vi "temperature_read.vi"(10 "T = Digital, F = Analog":bool) -> (3 "temperature array":dbl[](array[numeric]))   [LabVIEW 2021]
uses:
  <vilib>/DAQmx/read.llb/DAQmx Read (Analog 1D DBL NChan 1Samp).vi
  SmallBore_Labview/global_variables.vi
  <vilib>/DAQmx/create/channels.llb/DAQmx Create Channel (AI-Voltage-Basic).vi
  <vilib>/DAQmx/miscellaneous.llb/DAQmx Fill In Error Info.vi
panel:
  out "Thermometer 5: \nWater tank Small":dbl(slide) scale=0.0..100.0
  in  "Tab Control":enum32{"Digital", "Analog"}(tab)
  out "output array":bool[][](array[boolean])
  in  "Number of runs (>1)":i32=3
  in  "baud rate":u32=3906
  in  "No. expected bits":u16=64
  out "data":dbl[](array[numeric]) format="%0.2f"
  in  "milliseconds to wait":u32=100
  out "Thermometer 4: \nWater tank Big":dbl(slide) scale=0.0..100.0
  out "Thermometer 3: \nTx Filt Xfmer":dbl(slide) scale=0.0..100.0
  out "Thermometer 2: \nTx Filt L6":dbl(slide) scale=0.0..100.0
  out "Thermometer 1: \nTx Filt L7":dbl(slide) scale=0.0..100.0
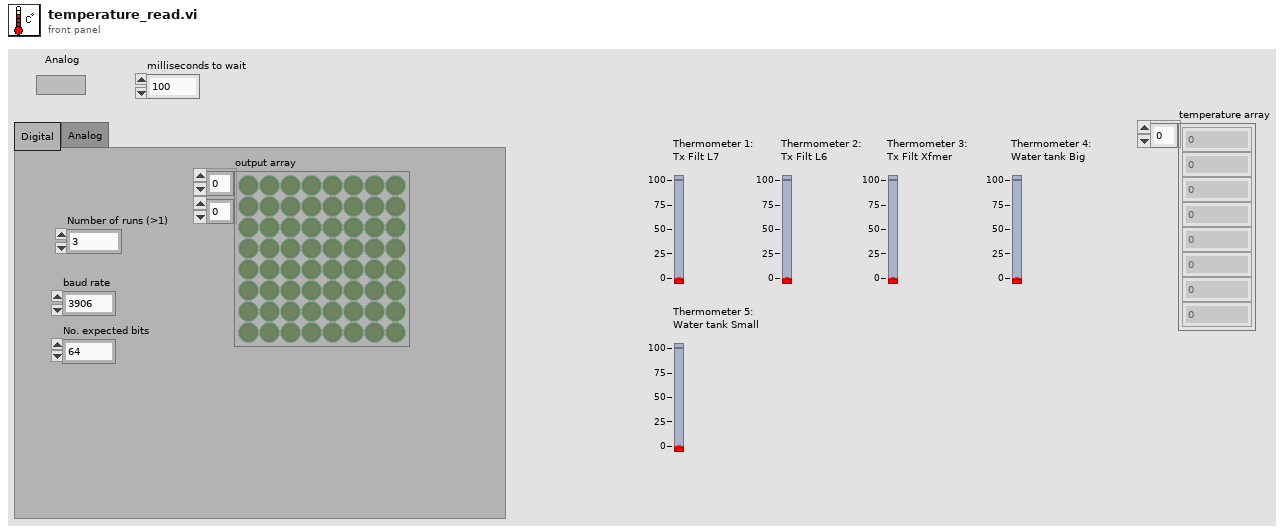
[diagram p1: front panel]
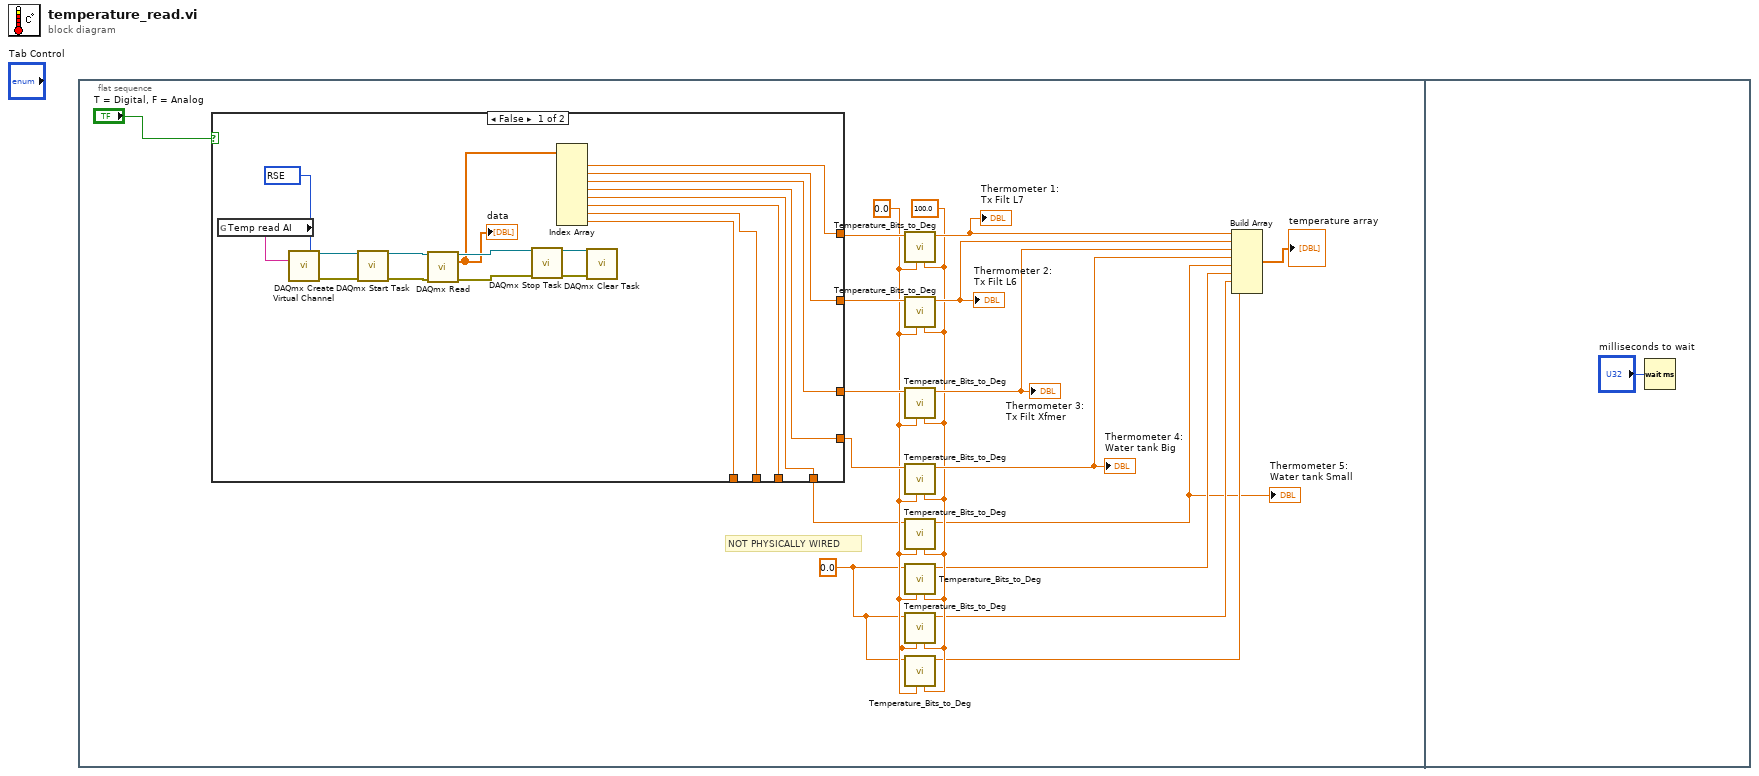
[diagram p0: block diagram]
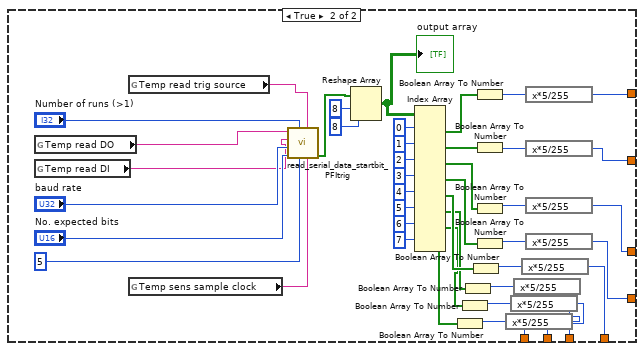
[diagram p2: hidden frame]
diagram:
  n1 = flat-sequence {
    frame #0 {
      w1 = 0.0 ("Val-In")
      w8 = 0.0 ("TMin")
      w7 = 100.0 ("TMax")
      # "NOT PHYSICALLY WIRED"
      n2 = case shown="False" "T = Digital, F = Analog" {
        tunnel: [w24 w51] -> w12
        tunnel: [w25 w53] -> w11
        tunnel: [w26 w55] -> w10
        tunnel: [w27 w56] -> w9
        tunnel: [w22 w48] -> w3
        tunnel: [w21 w40] -> _
        tunnel: [w20 w39] -> _
        tunnel: [w19 w38] -> _
        frame False {
          w23 = 10083 items=["Default"=-1, "RSE"=10083, "NRSE"=10078, "Differential"=10106, "Pseudodifferential"=12529] ("input terminal configuration")
          n3 = global read "global_variables.vi" "Temp read AI"() -> (w37:tag)
          n4 = call-poly <vilib>:"DAQmx Create Virtual Channel.vi"("input terminal configuration"=w23, "physical channels"=w37) -> ("task out"=w30:refnum<k21>, "error out"=w29:errorcluster)  [unwired: 12 in]
          n5 = call <vilib>:"DAQmx Start Task.vi"("task/channels in"=w30, "error in"=w29) -> ("task out"=w32:refnum<k21>, "error out"=w31:errorcluster)  [unwired: 12 in]
          n6 = call-poly <vilib>:"DAQmx Read.vi"("task/channels in"=w32, "error in"=w31) -> ("task out"=w34:refnum<k21>, "data"=w28:dbl[], "error out"=w33:errorcluster)  [unwired: 11 in]
          "data" <- w28
          n7 = call <vilib>:"DAQmx Stop Task.vi"("task/channels in"=w34, "error in"=w33) -> ("task out"=w36:refnum<k21>, "error out"=w35:errorcluster)  [unwired: 12 in]
          n8 = Index Array(array=w28) -> (element #1=w27:dbl, element #2=w26:dbl, element #3=w25:dbl, element #4=w24:dbl, element #5=w22:dbl, element #6=w21:dbl, element #7=w20:dbl, element #8=w19:dbl)  [unwired: 8 in]
          n9 = call <vilib>:"DAQmx Clear Task.vi"("task in"=w36, "error in"=w35) -> ()  [unwired: 13 in, 1 out]
        }
        frame True {
          n10 = global read "global_variables.vi" "Temp read DO"() -> (w75:tag)
          n11 = global read "global_variables.vi" "Temp read DI"() -> (w76:tag)
          n12 = global read "global_variables.vi" "Temp read trig source"() -> (w77:tag)
          n13 = global read "global_variables.vi" "Temp sens sample clock"() -> (w74:tag)
          n14 = call "read_serial_data_startbit_PFItrig.vi"("sample clock"=w74, "source"=w77, "samples per bit"=u16 5, "Number of runs"="Number of runs (>1)", "No. expected bits"="No. expected bits", "baud rate"="baud rate", "Digital input line"=w76, "Digital output line"=w75) -> ("output data LSB first"=w58:bool[])  [unwired: 2 in, 1 out]
          n15 = Reshape Array(w58, 8 ("dimension size"), 8 ("dimension size")) -> (w69:bool[][])
          "output array" <- w69
          n16 = Index Array(array=w69, index (row) #1=0 ("index (row)"), index (row) #2=1 ("index (row)"), index (row) #3=2 ("index (row)"), index (row) #4=3 ("index (row)"), index (row) #5=4 ("index (row)"), index (row) #6=5 ("index (row)"), index (row) #7=6 ("index (row)"), index (row) #8=7 ("index (row)")) -> (element #1=w70:bool[], element #2=w71:bool[], element #3=w72:bool[], element #4=w73:bool[], element #5=w47:bool[], element #6=w43:bool[], element #7=w42:bool[], element #8=w41:bool[])  [unwired: 8 in]
          n17 = Boolean Array To Number(Boolean array=w41) -> (number=w44:u32)
          n18 = Boolean Array To Number(Boolean array=w42) -> (number=w45:u32)
          n19 = Boolean Array To Number(Boolean array=w43) -> (number=w46:u32)
          n20 = Boolean Array To Number(Boolean array=w47) -> (number=w49:u32)
          n21 = Boolean Array To Number(Boolean array=w70) -> (number=w57:u32)
          n22 = Boolean Array To Number(Boolean array=w71) -> (number=w54:u32)
          n23 = Boolean Array To Number(Boolean array=w72) -> (number=w52:u32)
          n24 = Boolean Array To Number(Boolean array=w73) -> (number=w50:u32)
          n25 = expression code="x*5/255"(w44) -> (w38:u32)
          n26 = expression code="x*5/255"(w45) -> (w39:u32)
          n27 = expression code="x*5/255"(w46) -> (w40:u32)
          n28 = expression code="x*5/255"(w49) -> (w48:u32)
          n29 = expression code="x*5/255"(w57) -> (w56:u32)
          n30 = expression code="x*5/255"(w54) -> (w55:u32)
          n31 = expression code="x*5/255"(w52) -> (w53:u32)
          n32 = expression code="x*5/255"(w50) -> (w51:u32)
        }
      }
      n33 = call "Temperature_Bits_to_Deg.vi"("TMax"=w7, "TMin"=w8, "Val-In"=w9) -> ("TOut"=w18:dbl)  [unwired: 8 in]
      "Thermometer 1: \nTx Filt L7" <- w18
      n34 = call "Temperature_Bits_to_Deg.vi"("TMax"=w7, "TMin"=w8, "Val-In"=w10) -> ("TOut"=w17:dbl)  [unwired: 8 in]
      "Thermometer 2: \nTx Filt L6" <- w17
      n35 = call "Temperature_Bits_to_Deg.vi"("TMax"=w7, "TMin"=w8, "Val-In"=w11) -> ("TOut"=w16:dbl)  [unwired: 8 in]
      "Thermometer 3: \nTx Filt Xfmer" <- w16
      n36 = call "Temperature_Bits_to_Deg.vi"("TMax"=w7, "TMin"=w8, "Val-In"=w12) -> ("TOut"=w15:dbl)  [unwired: 8 in]
      "Thermometer 4: \nWater tank Big" <- w15
      n37 = call "Temperature_Bits_to_Deg.vi"("TMax"=w7, "TMin"=w8, "Val-In"=w3) -> ("TOut"=w2:dbl)  [unwired: 8 in]
      "Thermometer 5: \nWater tank Small" <- w2
      n38 = call "Temperature_Bits_to_Deg.vi"("TMax"=w7, "TMin"=w8, "Val-In"=w1) -> ("TOut"=w6:dbl)  [unwired: 8 in]
      n39 = call "Temperature_Bits_to_Deg.vi"("TMax"=w7, "TMin"=w8, "Val-In"=w1) -> ("TOut"=w5:dbl)  [unwired: 8 in]
      n40 = call "Temperature_Bits_to_Deg.vi"("TMax"=w7, "TMin"=w8, "Val-In"=w1) -> ("TOut"=w4:dbl)  [unwired: 8 in]
      n41 = Build Array(w18, w17, w16, w15, w2, w6, w5, w4) -> (→"temperature array":dbl[])
    }
    frame #1 {
      n42 = Wait (ms)(milliseconds to wait="milliseconds to wait") -> ()  [unwired: 1 out]
    }
  }
